vi "SetpointsToTCP.vi"(10 "remote port or service name":u16=10001, 11 "address":string="192.168.1.11") -> (0 "error out":errorcluster, 3 "TCP Connected?":bool)   [LabVIEW 2011]
uses:
  2-RIO/2 Typedefs/setpoints to boat.ctl
  2-RIO/2 Typedefs/sail setpt.ctl
  2-RIO/2 Typedefs/rudder angle.ctl
  2-RIO/2 Typedefs/generalized actuator status.ctl
  2-RIO/2 Typedefs/indicator LED.ctl
  2-RIO/2 Globals/2 Global.vi
panel:
  out "output array":T1[](array[typedef])
  out "Setpoints to boat out":T2
  in  "VI Stop":bool
  # "This is the Set-Points to TCP writer.\n\nThis vi reads the global variable setpoints and passes them through to the TCP connection.\n\nTODO: make it actually work. Connection to the global variable seems a bit glitchy, as does the TCP connection."
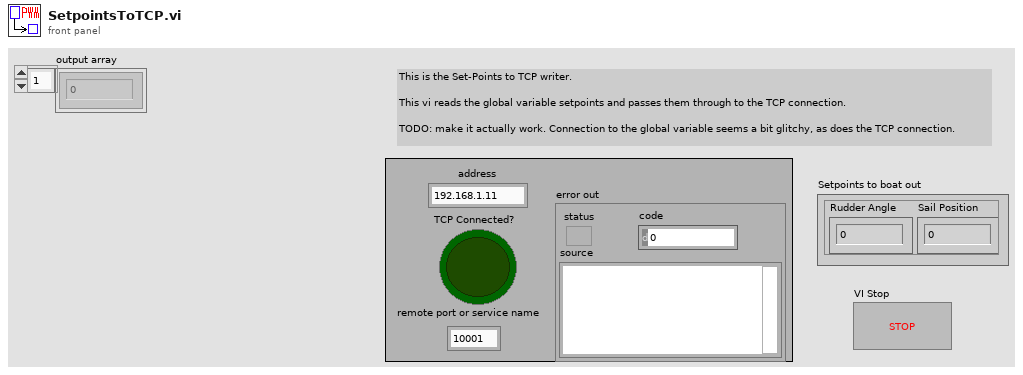
[diagram p1: front panel]
types:
  T1 = typedef "rudder angle.ctl" = dbl
  T2 = typedef "setpoints to boat.ctl" = cluster{"Sail Position":T3, "Rudder Angle":T1}
  T3 = typedef "sail setpt.ctl" = dbl
  T4 = typedef "generalized actuator status.ctl" = cluster{"Actuator Connected":T5}
  T5 = typedef "indicator LED.ctl" = bool
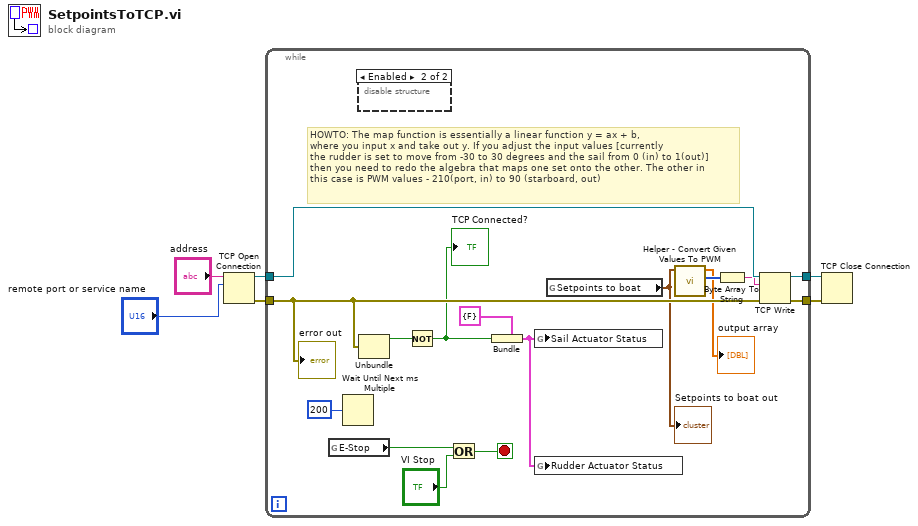
[diagram p0: block diagram]
diagram:
  n1 = TCP Open Connection(address="address", remote port or service name="remote port or service name") -> (connection ID=w2:refnum<k5>, error out=w4:errorcluster)  [unwired: 3 in]
  n2 = while {
    tunnel: w4 -> [w19]
    tunnel: [w22] -> w3
    tunnel: w2 -> [w21]
    tunnel: [w20] -> w1
    stop <- w15 stop-if-true
    # "HOWTO: The map function is essentially a linear function y = ax + b,\nwhere you input x and take out y. If you adjust the input values [currently\nthe rudder is set to move from -30 to 30 degrees and the sail from 0 (in) to 1(out)]\nthen you need to redo the algebra that maps one set onto the other. The other in\nthis case is PWM values - 210(port, in) to 90 (starboard, out)"
    n3 = global read "2 Global.vi" "E-Stop"() -> (w13:bool)
    n4 = Wait Until Next ms Multiple(millisecond multiple=u32 200) -> ()  [unwired: 1 out]
    n5 = disable-structure shown="Enabled" {
      frame Disabled {
      }
      frame Enabled {
      }
    }
    n6 = Unbundle(w19) -> ("status"=w18:bool)  [unwired: 2 out]
    n7 = Not(x=w18) -> (.not. x?=w11:bool)
    "TCP Connected?" <- w11
    n8 = Or(x=w13, y="VI Stop") -> (x .or. y?=w15:bool)
    n9 = Bundle(cluster=T4 {"Actuator Connected"=FALSE} ("Sail Actuator Status"), "Actuator Connected"=w11) -> (w10:T4)
    n10 = global write "2 Global.vi" "Sail Actuator Status"(w10) -> ()
    n11 = global write "2 Global.vi" "Rudder Actuator Status"(w10) -> ()
    n12 = global read "2 Global.vi" "Setpoints to boat"() -> (w7:T2)
    "Setpoints to boat out" <- w7
    n13 = call "Helper - Convert Given Values To PWM.vi"("Setpoints to boat"=w7) -> ("Array"=w9:u8[], "output array"=→"output array":T1[])  [unwired: 9 in]
    n14 = Byte Array To String(unsigned byte array=w9) -> (string=w17:string)
    n15 = TCP Write(connection ID=w21, data in=w17, error in (no error)=w19) -> (connection ID out=w20:refnum<k5>, error out=w22:errorcluster)  [unwired: 1 in, 1 out]
    "error out" <- w19
  }
  n16 = TCP Close Connection(connection ID=w1, error in (no error)=w3) -> ()  [unwired: 1 in, 2 out]
